vi "EmergencyAlarm.vi"() -> (0 "error out":errorcluster, 3 "复位":bool)   [LabVIEW 2011]
uses:
  Global Variable.vi
  Global System.vi
panel:
  in  "stop":bool
  # "EMERGENCY!"
  # "1、Please check hardware!"
  # "2、Release Emergency Button!"
  # "3、Click Reset Button!"
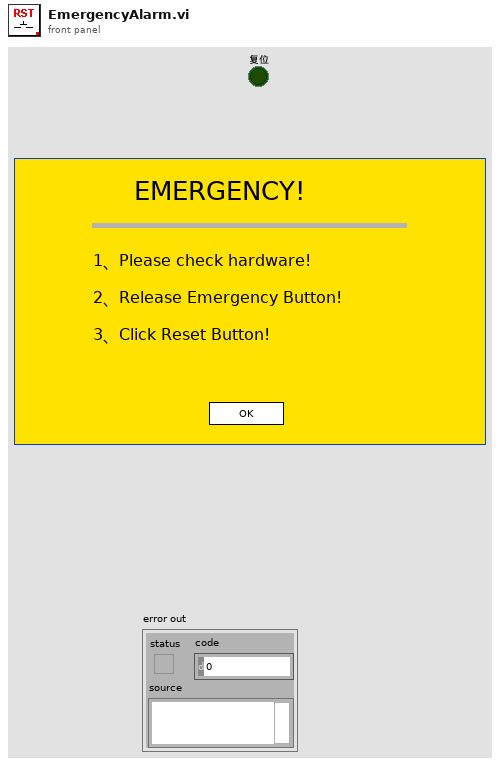
[diagram p1: front panel]
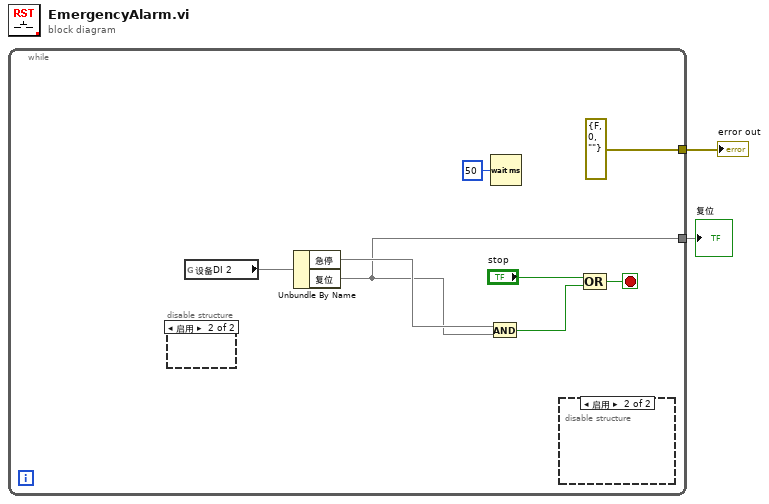
[diagram p0: block diagram]
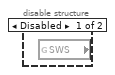
[diagram p2: hidden frame]
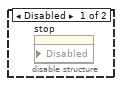
[diagram p3: hidden frame]
diagram:
  n1 = while {
    tunnel: [errorcluster {"status"=FALSE, "code"=0, "source"=""} ("sys error")] -> w2
    tunnel: [w3] -> w1
    stop <- w10 stop-if-true
    n2 = disable-structure shown="启用" {
      frame Disabled {
        n3 = global read "Global Variable.vi" "SWS"() -> ()  [unwired: 1 out]
      }
      frame Enabled {
      }
    }
    n4 = global read "Global System.vi" "设备DI 2"() -> (w5)
    n5 = Unbundle By Name(w5) -> ("急停"=w4, "复位"=w3)
    n6 = And(x=w4, y=w3) -> (x .and. y?=w7:bool)
    n7 = Wait (ms)(milliseconds to wait=u32 50) -> ()  [unwired: 1 out]
    n8 = disable-structure shown="启用" {
      frame Disabled {
        n9 = property on="stop" class="Bool" props=["Disabled"]() -> ()  [unwired: 3 in, 2 out]
      }
      frame Enabled {
      }
    }
    n10 = Compound Arithmetic op=OR("stop", w7) -> (w10:bool)
  }
  "error out" <- w2
  "复位" <- w1
